vi "Adjust Cell to Write Measurement.vi"(8 "error in (no error)":errorcluster, 10 "Incremento":i32, 11 "Ini File Output in":T1) -> (0 "error out":errorcluster, 3 "Ini File Output out":T1)   [LabVIEW 2015]
doc: "VI usada para indicar as Células onde serão escritos as medições."
uses:
  controls/Ini File Output.ctl
  <vilib>/addons/_office/NI_ReportGenerationToolkit.lvlib
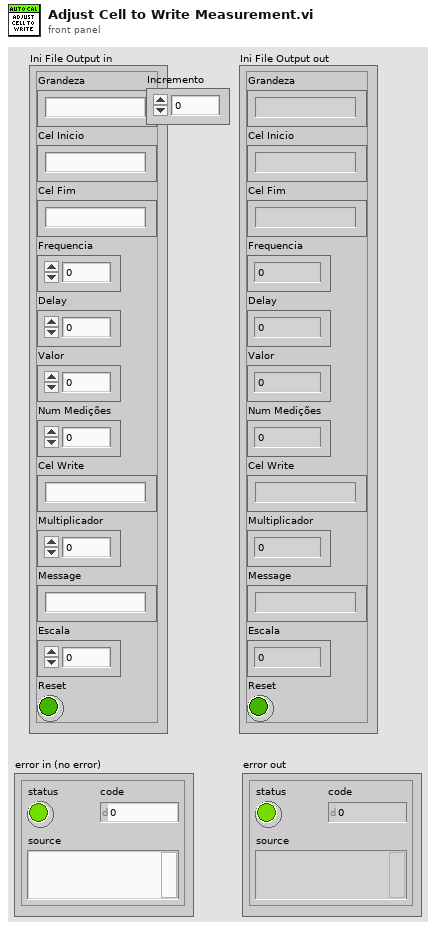
[diagram p1: front panel]
types:
  T1 = typedef "Ini File Output.ctl" = cluster{"Grandeza":string, "Cel Inicio":string, "Cel Fim":string, "Frequencia":dbl, "Delay":dbl, "Valor":dbl, "Num Medições":i32, "Cel Write":string, "Multiplicador":dbl, "Message":string, "Escala":dbl, "Reset":bool}
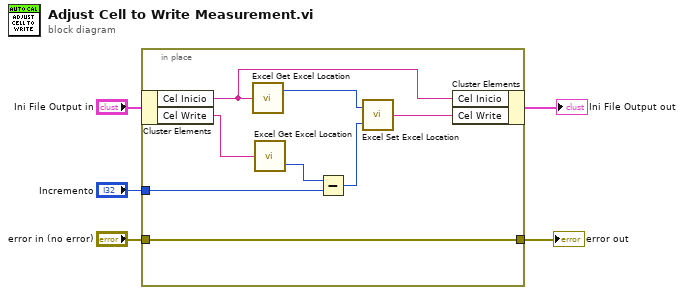
[diagram p0: block diagram]
diagram:
  n1 = in-place {
    in-place-border: "error in (no error)" -> [w13]
    in-place-border: [w13] -> w5
    in-place-border: "Incremento" -> [w6]
    n2 = in-place-cluster #1("Ini File Output in") -> ("Cel Inicio"=w11:string, "Cel Write"=w12:string)
    n3 = call <vilib>:"Excel Get Excel Location.vi"("cell's name"=w11) -> ("row"=w8:i32)  [unwired: 1 out]
    n4 = call <vilib>:"Excel Get Excel Location.vi"("cell's name"=w12) -> ("column"=w7:i32)  [unwired: 1 out]
    n5 = Subtract(x=w7, y=w6) -> (x-y=w10:i32)
    n6 = call <vilib>:"Excel Set Excel Location.vi"("column"=w10, "row"=w8) -> ("cell's name"=w9:string)
    n7 = in-place-cluster #1("Cel Inicio"=w11, "Cel Write"=w9) -> (→"Ini File Output out":T1)
  }
  "error out" <- w5
